vi "VNARP-VNASETTING CLTR MANAGMENT.vi"(2 "VNA SETTING CLUSTER":T1 {"SPACING 2" min=0.0 max=100.0 step=0.5; "Points N° 2" min=0 max=100 step=1; "PROBE" min=0.0 max=100.0 step=0.5; "PUMP" min=0.0 max=100.0 step=0.5}, 3 "RP VNA SETTING":T2={"F start"=200000, "F stop"=2000000, "Sweep size"=2000, "Decimation"=5000, "F_corr"=0, "Ph_OUT1"=0, "Ph_OUT2"=0, "OUT_Lvl1"=32700, "OUT_Lvl2"=32700, "GPIO"=0}) -> (1 "OUTPUT VNA SETTINGS":T2)   [LabVIEW 2021]
uses:
  Channel parameters.ctl
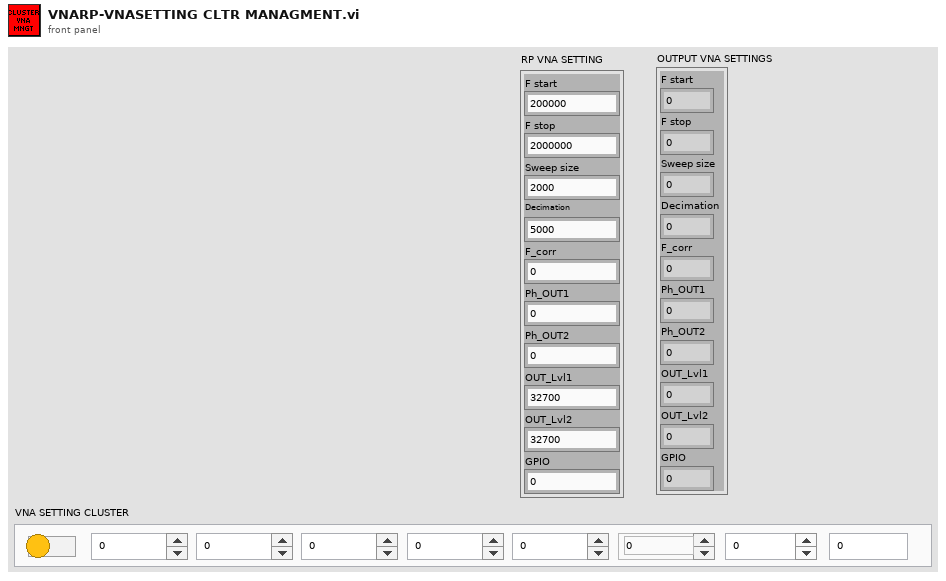
[diagram p1: front panel]
types:
  T1 = typedef "Channel parameters.ctl" = cluster{"START 2":dbl, "STOP 2":dbl, "CENTER 2":dbl, "SPAN 2":dbl, "CHANNEL TRACK ?":bool, "PUMP":dbl, "PROBE":dbl, "Points N° 2":i32, "SPACING 2":dbl}
  T2 = cluster{"F start":u32, "F stop":u32, "Sweep size":u32, "Decimation":u32, "F_corr":u32, "Ph_OUT1":u32, "Ph_OUT2":u32, "OUT_Lvl1":u32, "OUT_Lvl2":u32, "GPIO":u32}
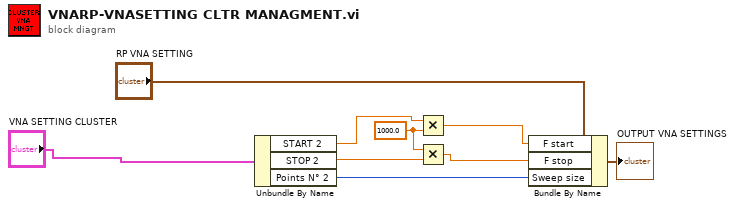
[diagram p0: block diagram]
diagram:
  w8 = 1000.0 ("y")
  n1 = Unbundle By Name("VNA SETTING CLUSTER") -> ("START 2"=w7:dbl, "STOP 2"=w6:dbl, "Points N° 2"=w3:i32)
  n2 = Multiply(x=w7, y=w8) -> (x*y=w4:dbl)
  n3 = Multiply(x=w8, y=w6) -> (x*y=w5:dbl)
  n4 = Bundle By Name(cluster="RP VNA SETTING", "F start"=w4, "F stop"=w5, "Sweep size"=w3) -> (→"OUTPUT VNA SETTINGS":T2)
